vi "WiiMote Read BalanceBoard.vi"(0 "BalanceBoardState":refnum<k24>, 11 "error in":errorcluster) -> (4 "Balance Board State":T1, 15 "error out":errorcluster)   [LabVIEW 2011]
uses:
  D:/jjensen/Documents/Lab Book/embeddedLab/exercises/LabVIEW/.WiiMote/Dependencies/WiimoteLib.dll
  .WiiMote/Dependencies/WiimoteLib.dll
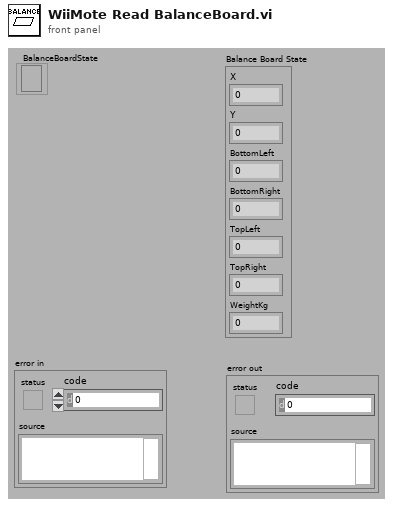
[diagram p1: front panel]
types:
  T1 = cluster{"X":sgl, "Y":sgl, "BottomLeft":sgl, "BottomRight":sgl, "TopLeft":sgl, "TopRight":sgl, "WeightKg":sgl}
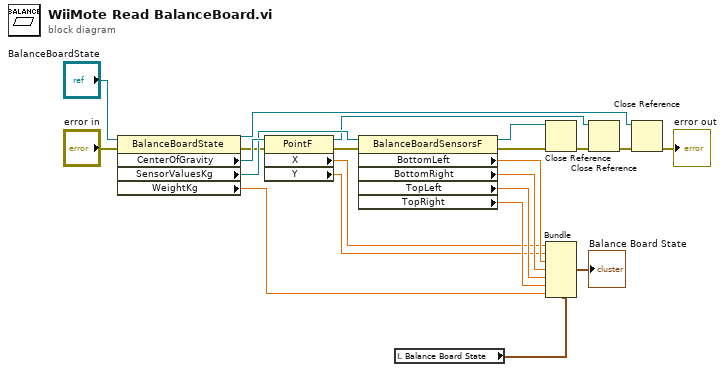
[diagram p0: block diagram]
diagram:
  n1 = property class="BalanceBoardState"(reference="BalanceBoardState", error in="error in") -> (reference out=w8:refnum<k24>, error out=w6:errorcluster, "CenterOfGravity"=w14:refnum<k24>, "SensorValuesKg"=w13:refnum<k24>, "WeightKg"=w21:sgl)
  n2 = property class="PointF"(reference=w14, error in=w6) -> (reference out=w9:refnum<k24>, error out=w5:errorcluster, "X"=w15:sgl, "Y"=w16:sgl)
  n3 = property class="BalanceBoardSensorsF"(reference=w13, error in=w5) -> (reference out=w10:refnum<k24>, error out=w7:errorcluster, "BottomLeft"=w17:sgl, "BottomRight"=w18:sgl, "TopLeft"=w19:sgl, "TopRight"=w20:sgl)
  n4 = local read "Balance Board State"() -> (w1:T1)
  n5 = Close Reference(reference=w10, error in (no error)=w7) -> (error out=w4:errorcluster)
  n6 = Bundle(cluster=w1, "X"=w15, "Y"=w16, "BottomLeft"=w17, "BottomRight"=w18, "TopLeft"=w19, "TopRight"=w20, "WeightKg"=w21) -> (→"Balance Board State":T1)
  n7 = Close Reference(reference=w9, error in (no error)=w4) -> (error out=w3:errorcluster)
  n8 = Close Reference(reference=w8, error in (no error)=w3) -> (error out=→"error out":errorcluster)
